vi "Read Flow Rate.vi"(8 "error in":errorcluster, 10 "listen period":sgl=0.1, 11 "Brooks MFC in":refnum<class "Brooks MFC.lvclass">) -> (0 "error out":errorcluster, 1 "units":string="Liters/minute", 2 "flow rate":sgl, 3 "Brooks MFC out":refnum<class "Brooks MFC.lvclass">)   [LabVIEW 2016, in "Brooks MFC.lvclass"]
uses:
  Brooks MFC.lvclass
  Brooks MFC.lvclass/Brooks MFC.ctl
  Instance           1 22Saved   Read Flow Rate .vi
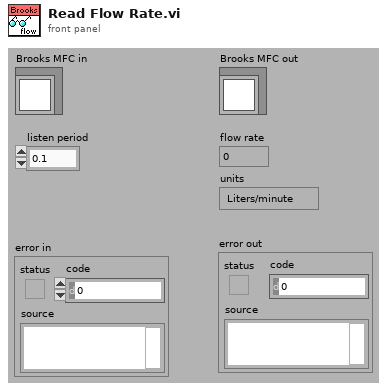
[diagram p1: front panel]
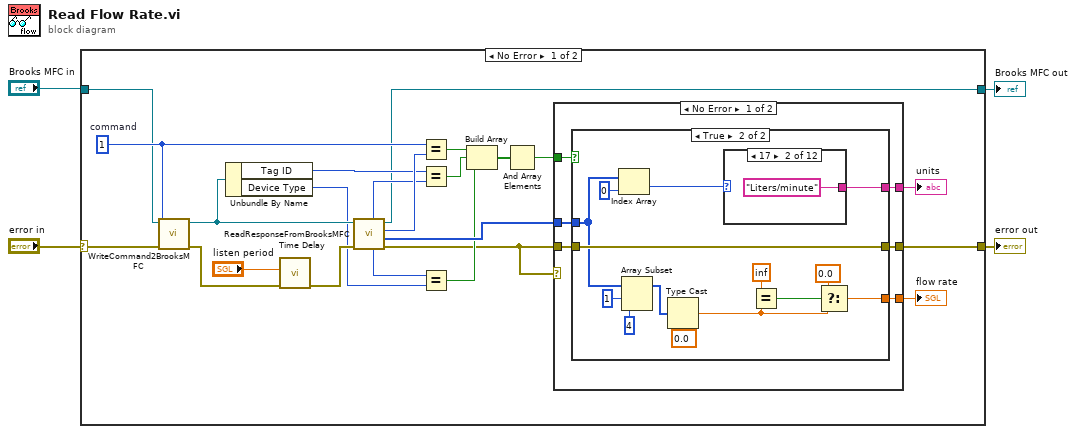
[diagram p0: block diagram]
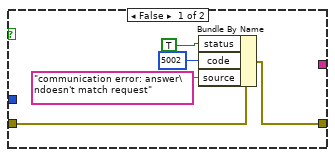
[diagram p2: hidden frame]
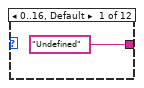
[diagram p3: hidden frame]
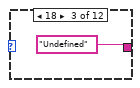
[diagram p4: hidden frame]
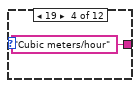
[diagram p5: hidden frame]
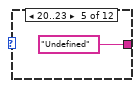
[diagram p6: hidden frame]
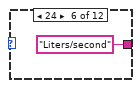
[diagram p7: hidden frame]
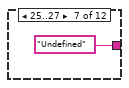
[diagram p8: hidden frame]
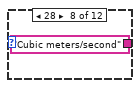
[diagram p9: hidden frame]
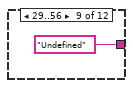
[diagram p10: hidden frame]
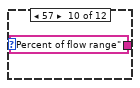
[diagram p11: hidden frame]
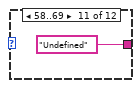
[diagram p12: hidden frame]
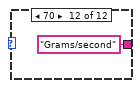
[diagram p13: hidden frame]
diagram:
  n1 = case shown="No Error" "error in" {
    selector: "error in" -> [w10 w67]
    tunnel: [w9 w67] -> w2
    tunnel: "Brooks MFC in" -> [w8 w66]
    tunnel: [w5 w66] -> w1
    frame No Error {
      w13 = u8 1  # command
      n2 = call "WriteCommand2BrooksMFC.vi"("error in"=w10, "Command"=w13, "Brooks MFC in"=w8) -> ("error out"=w23:errorcluster, "Brooks MFC out"=w11:refnum<class "Brooks MFC.lvclass">)  [unwired: 6 in, 1 out]
      n3 = Unbundle By Name(w11) -> ("Tag ID"=w6:u32, "Device Type"=w7:u8)
      n4 = call "Time Delay"("error in (no error)"=w23, "Delay Time (s)"="listen period") -> ("error out"=w21:errorcluster)  [unwired: 9 in]
      n5 = call "ReadResponseFromBrooksMFC.vi"("error in"=w21, "Brooks MFC in"=w11) -> ("error out"=w12:errorcluster, "Data"=w27:u8[], "Command"=w24:u8, "Brooks MFC out"=w5:refnum<class "Brooks MFC.lvclass">, "device type"=w19:u8, "tag ID"=w20:u32)  [unwired: 4 in]
      n6 = Equal?(x=w13, y=w24) -> (x = y?=w18:bool)
      n7 = Equal?(x=w6, y=w20) -> (x = y?=w17:bool)
      n8 = Equal?(x=w19, y=w7) -> (x = y?=w16:bool)
      n9 = Build Array(w18, w17, w16) -> (w15:bool[])
      n10 = And Array Elements(Boolean array=w15) -> (logical AND=w14:bool)
      n11 = case shown="No Error" w12 {
        tunnel: w12 -> [w33 w65]
        tunnel: w27 -> [w32 _]
        tunnel: [w31 w65] -> w9
        tunnel: [w30 _] -> w26
        tunnel: [w29 _] -> w25
        tunnel: w14 -> [w28 _]
        frame No Error {
          n12 = case shown="True" w28 {
            tunnel: w32 -> [_ w49]
            tunnel: w33 -> [w35 w50]
            tunnel: [w34 w50] -> w31
            tunnel: [_ w47] -> w29
            tunnel: [_ w43] -> w30
            frame False {
              n13 = Bundle By Name(cluster=w35, "status"=TRUE ("Bundle Element"), "code"=5002 ("Bundle Element"), "source"="communication error: answer\ndoesn't match request" ("Bundle Element")) -> (w34:errorcluster)
            }
            frame True {
              n14 = Index Array(array=w49, index=0 ("Index")) -> (element=w42:u8)
              n15 = Array Subset(array=w49, index=1 ("Array Index"), length=4 ("Array Length")) -> (w41:u8[])
              n16 = Type Cast(type=sgl 0.0 ("x"), x=w41) -> (*(type *) &x=w39:sgl)
              n17 = case shown="17" w42 {
                tunnel: ["Undefined" "Liters/minute" "Undefined" "Cubic meters/hour" "Undefined" "Liters/second" "Undefined" "Cubic meters/second" "Undefined" "Percent of flow range" "Undefined" "Grams/second"] -> w47
                frame 0..16, Default {
                }
                frame 17 {
                }
                frame 18 {
                }
                frame 19 {
                }
                frame 20..23 {
                }
                frame 24 {
                }
                frame 25..27 {
                }
                frame 28 {
                }
                frame 29..56 {
                }
                frame 57 {
                }
                frame 58..69 {
                }
                frame 70 {
                }
              }
              n18 = Equal?(x=sgl inf ("Single"), y=w39) -> (x = y?=w45:bool)
              n19 = Select(t=sgl 0.0 ("x"), s=w45, f=w39) -> (s? t:f=w43:sgl)
            }
          }
        }
        frame Error {
        }
      }
      "units" <- w25
      "flow rate" <- w26
    }
    frame Error {
    }
  }
  "error out" <- w2
  "Brooks MFC out" <- w1
